vi "csvFileExplorer.vi"() -> ()   [LabVIEW 2019]
uses:
  <vilib>/Math Plots/3D Math Plots/3D Surface/3D Surface XCtrl/3D Surface.xctl
  <vilib>/Utility/file.llb/Read Delimited Spreadsheet (string).vi
  <vilib>/Math Plots/3D Math Plots/3D Surface/3D Surface Datatype/Public/Plot Helper (Vector).vi
  <vilib>/Analysis/NI_AALBase.lvlib
  <vilib>/Math Plots/3D Math Plots/3D Surface/3D Surface Datatype/3D Surface Datatype.lvclass
panel:
  out "Intensity Graph 2":i32[][](graph)
  in  "file path (dialog if empty)":path
  out "Detector Surface 2":refnum<class "3D Plot Datatype.lvclass">[](xcontrol)
  out "Noisy Pixel List":i32[][](array[numeric])
  out "all rows":string[][](array[string])
  out "Intensity Graph":u32[][](graph)
  out "Detector Surface":refnum<class "3D Plot Datatype.lvclass">[](xcontrol)
  out "Event Count Histogram":T1(graph)
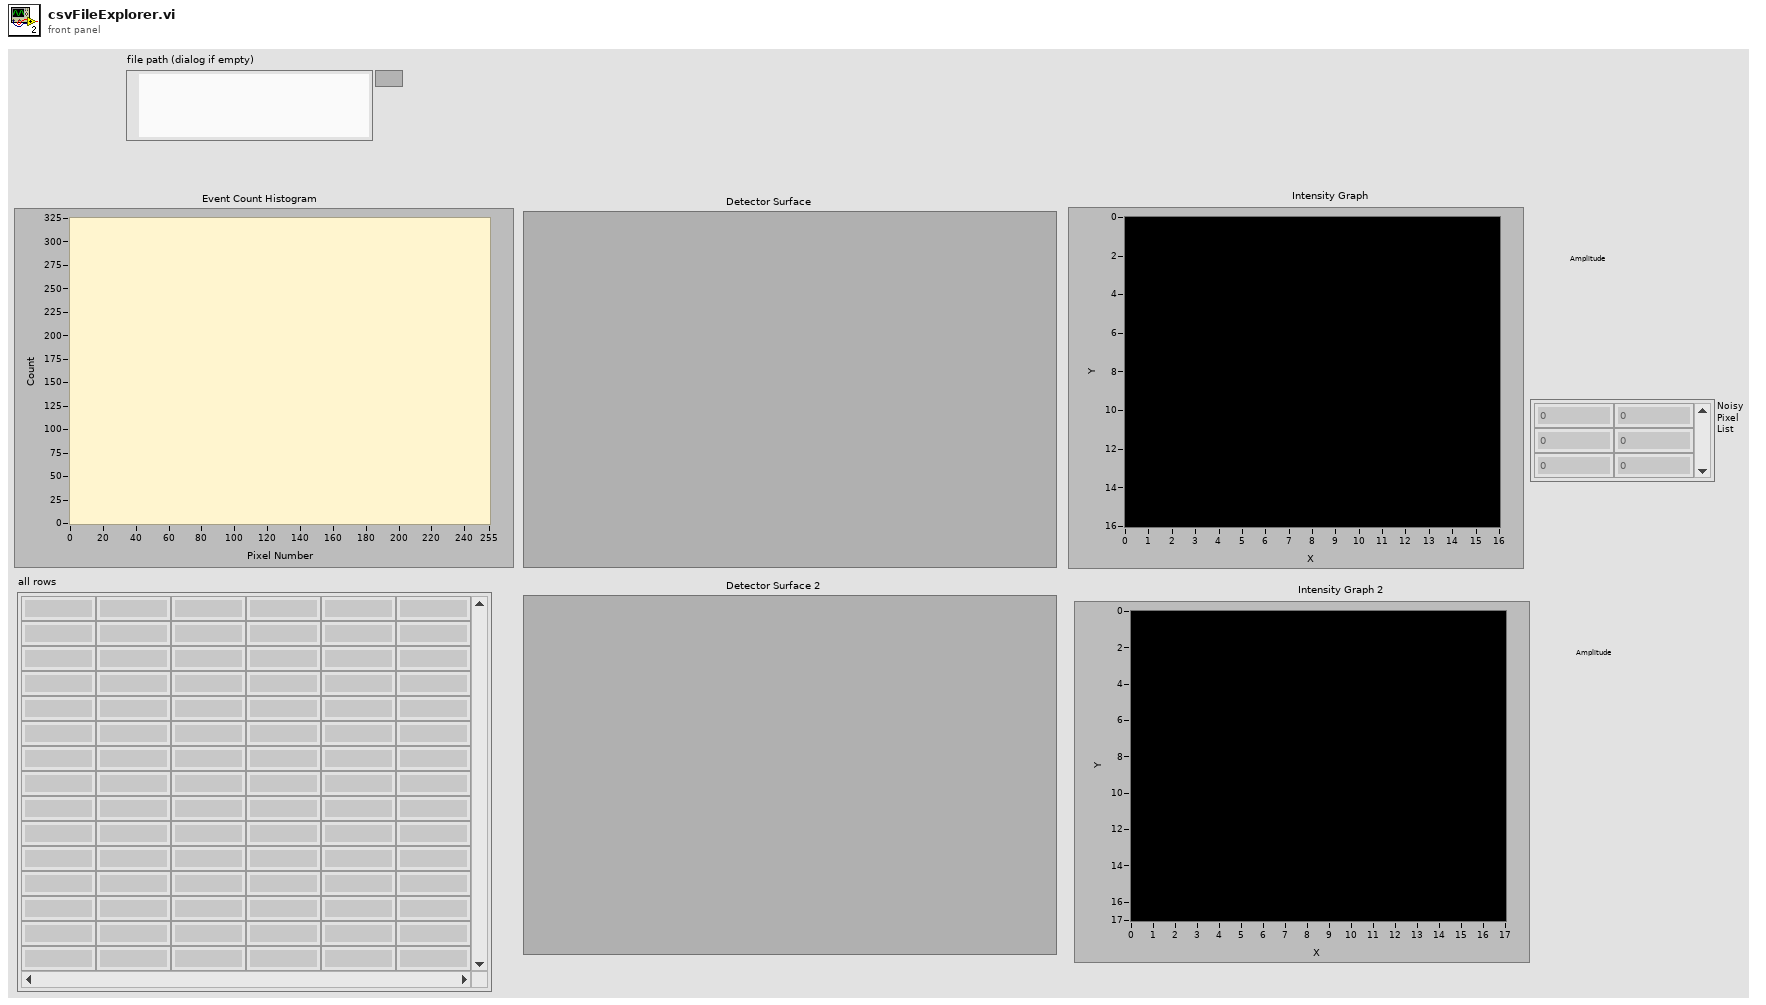
[diagram p1: front panel]
types:
  T1 = cluster{"X Values":dbl[], "Histogram: h(x)":i32[]}
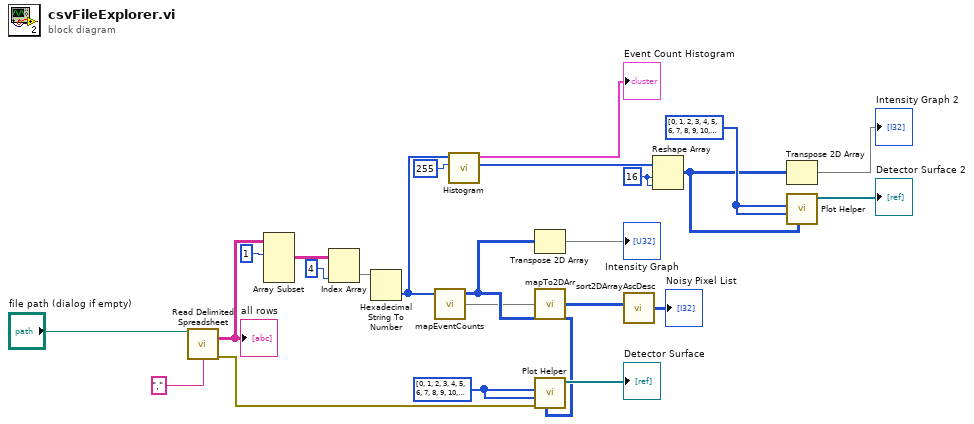
[diagram p0: block diagram]
diagram:
  w4 = u8[] [0, 1, 2, 3, 4, 5, 6, 7, 8, 9, 10, 11, 12, 13, 14, 15, 0, 1, 2, 3, 4, 5, 6, 7, 8, 9, 10, 11, 12, 13, 14, 15, 0, 1, 2, 3, 4, 5, 6, 7, 8, 9, 10, 11, 12, 13, 14, 15, 0, 1, 2, 3, 4, 5, 6, 7, 8, 9, 10, 11, 12, 13, 14, 15, 0, 1, 2, 3, 4, 5, 6, 7, 8, 9, 10, 11, 12, 13, 14, 15, 0, 1, 2, 3, 4, 5, 6, 7, 8, 9, 10, 11, 12, 13, 14, 15, 0, 1, 2, 3, 4, 5, 6, 7, 8, 9, 10, 11, 12, 13, 14, 15, 0, 1, 2, 3, 4, 5, 6, 7, 8, 9, 10, 11, 12, 13, 14, 15, 0, 1, 2, 3, 4, 5, 6, 7, 8, 9, 10, 11, 12, 13, 14, 15, 0, 1, 2, 3, 4, 5, 6, 7, 8, 9, 10, 11, 12, 13, 14, 15, 0, 1, 2, 3, 4, 5, 6, 7, 8, 9, 10, 11, 12, 13, 14, 15, 0, 1, 2, 3, 4, 5, 6, 7, 8, 9, 10, 11, 12, 13, 14, 15, 0, 1, 2, 3, 4, 5, 6, 7, 8, 9, 10, 11, 12, 13, 14, 15, 0, 1, 2, 3, 4, 5, 6, 7, 8, 9, 10, 11, 12, 13, 14, 15, 0, 1, 2, 3, 4, 5, 6, 7, 8, 9, 10, 11, 12, 13, 14, 15, 0, 1, 2, 3, 4, 5, 6, 7, 8, 9, 10, 11, 12, 13, 14] ("Array")
  w5 = 16 ("dimension size")
  w8 = u8[] [0, 1, 2, 3, 4, 5, 6, 7, 8, 9, 10, 11, 12, 13, 14, 15, 0, 1, 2, 3, 4, 5, 6, 7, 8, 9, 10, 11, 12, 13, 14, 15, 0, 1, 2, 3, 4, 5, 6, 7, 8, 9, 10, 11, 12, 13, 14, 15, 0, 1, 2, 3, 4, 5, 6, 7, 8, 9, 10, 11, 12, 13, 14, 15, 0, 1, 2, 3, 4, 5, 6, 7, 8, 9, 10, 11, 12, 13, 14, 15, 0, 1, 2, 3, 4, 5, 6, 7, 8, 9, 10, 11, 12, 13, 14, 15, 0, 1, 2, 3, 4, 5, 6, 7, 8, 9, 10, 11, 12, 13, 14, 15, 0, 1, 2, 3, 4, 5, 6, 7, 8, 9, 10, 11, 12, 13, 14, 15, 0, 1, 2, 3, 4, 5, 6, 7, 8, 9, 10, 11, 12, 13, 14, 15, 0, 1, 2, 3, 4, 5, 6, 7, 8, 9, 10, 11, 12, 13, 14, 15, 0, 1, 2, 3, 4, 5, 6, 7, 8, 9, 10, 11, 12, 13, 14, 15, 0, 1, 2, 3, 4, 5, 6, 7, 8, 9, 10, 11, 12, 13, 14, 15, 0, 1, 2, 3, 4, 5, 6, 7, 8, 9, 10, 11, 12, 13, 14, 15, 0, 1, 2, 3, 4, 5, 6, 7, 8, 9, 10, 11, 12, 13, 14, 15, 0, 1, 2, 3, 4, 5, 6, 7, 8, 9, 10, 11, 12, 13, 14, 15, 0, 1, 2, 3, 4, 5, 6, 7, 8, 9, 10, 11, 12, 13, 14] ("Array")
  n1 = call-poly <vilib>:"Read Delimited Spreadsheet.vi"("file path (dialog if empty)"="file path (dialog if empty)", "delimiter (\\t)"=",") -> ("all rows"=w23:string[][], "error out"=w14:errorcluster)  [unwired: 8 in, 4 out]
  "all rows" <- w23
  n2 = Array Subset(array=w23, index (row)=1 ("index")) -> (w21:string[][])  [unwired: 3 in]
  n3 = Index Array(array=w21, index (col)=4 ("disabled index (col)")) -> (element=w19:string[])  [unwired: 1 in]
  n4 = Hexadecimal String To Number(string=w19) -> (number=w17:u32[])  [unwired: 2 in, 1 out]
  n5 = call "mapEventCounts.vi"("Count"=w17) -> ("Counts (map)"=w9:map{u32, u32}, "Count Grid"=w13:u32[][])  [unwired: 3 in]
  n6 = call <vilib>:"Histogram.vi"("intervals"=255, "X"=w17) -> ("Histogram: h(x)"=w6:i32[], "Histogram Graph"=→"Event Count Histogram":T1)  [unwired: 5 in, 3 out]
  n7 = Transpose 2D Array(2D array=w13) -> (transposed array=→"Intensity Graph":u32[][])
  n8 = call "mapTo2DArr.vi"("Map"=w9) -> ("2D Array"=w10:i32[][])
  n9 = call-poly <vilib>:"Plot Helper.vi"("z matrix"=w13, "error in (no error)"=w14, "y vector"=w8, "x vector"=w8) -> ("3D Plot lvclass Array out"=→"Detector Surface":refnum<class "3D Plot Datatype.lvclass">[])  [unwired: 2 in, 5 out]
  n10 = call "sort2DArrayAscDesc.vi"("2D Array"=w10) -> ("sorted 2D array"=→"Noisy Pixel List":i32[][])  [unwired: 5 in]
  n11 = Reshape Array(w6, w5, w5) -> (w2:i32[][])
  n12 = Transpose 2D Array(2D array=w2) -> (transposed array=→"Intensity Graph 2":i32[][])
  n13 = call-poly <vilib>:"Plot Helper.vi"("z matrix"=w2, "y vector"=w4, "x vector"=w4) -> ("3D Plot lvclass Array out"=→"Detector Surface 2":refnum<class "3D Plot Datatype.lvclass">[])  [unwired: 3 in, 5 out]
